vi "TCPIP GUID Lookup.vi"() -> ()   [LabVIEW 2013, in "TCPIP Custom Device.lvlib"]
doc: "Use this Global VI to access the GUIDs assigned to the page resources of the Custom Device."
uses:
  TCPIP Custom Device.lvlib
panel:
  in  "Custom Device":string="8a313c66-5fc7-4697-8af5-eed800caa9aa"
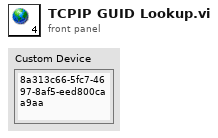
[diagram p1: front panel]
diagram:
